vi "Fired.vi"(8 "error in (no error)":errorcluster, 11 "module in":refnum<class "CRON.lvclass">) -> (0 "error out":errorcluster, 3 "module out":refnum<class "CRON.lvclass">)   [LabVIEW 2024, in "CRON.lvclass"]
uses:
  CRON.lvclass
  CRON.lvclass/CRON.ctl
  C:/Git/JA/JQMH/RQMHCore/ModuleCore/Module.lvclass
  C:/Git/JA/JQMH/ModuleTemplates/CRON/CRON.lvclass
  RQMHCore/ModuleCore/Module.lvclass
  Fired.ctl
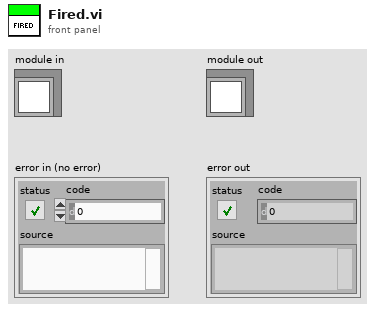
[diagram p1: front panel]
types:
  T1 = typedef "CRON.lvclass/Fired.ctl" = cluster{"Module":refnum<class "Module.lvclass">}
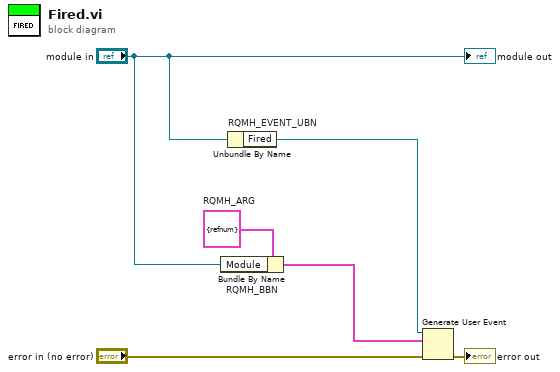
[diagram p0: block diagram]
diagram:
  w3 = T1 {"Module"=refnum}  # RQMH_ARG
  n1 = Bundle By Name "RQMH_BBN"(cluster=w3, "Module"="module in") -> (w2:T1)
  n2 = Unbundle By Name "RQMH_EVENT_UBN"("module in") -> ("Fired"=w6:refnum<user-event>)
  n3 = Generate User Event(user event=w6, event data cluster=w2, error in="error in (no error)") -> (error out=→"error out":errorcluster)  [unwired: 1 in, 1 out]
  "module out" <- "module in"
